vi "Timer Status.vi"(8 "error in":errorcluster, 9 "Position Correct?":bool, 10 "Step Status":string, 11 "Car Wash Steps":string[][](array[string])) -> (0 "error out":errorcluster, 2 "Timer Control":T1=enum."Start", 3 "Time Target":dbl, 5 "New Step Status":string)   [LabVIEW 2020]
uses:
  Timer Controls.ctl
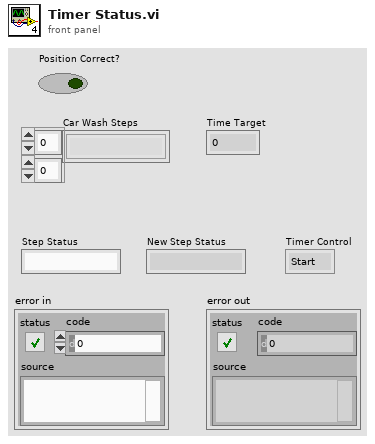
[diagram p1: front panel]
types:
  T1 = typedef "Timer Controls.ctl" = enum16{"Reset", "Start", "Stop"}
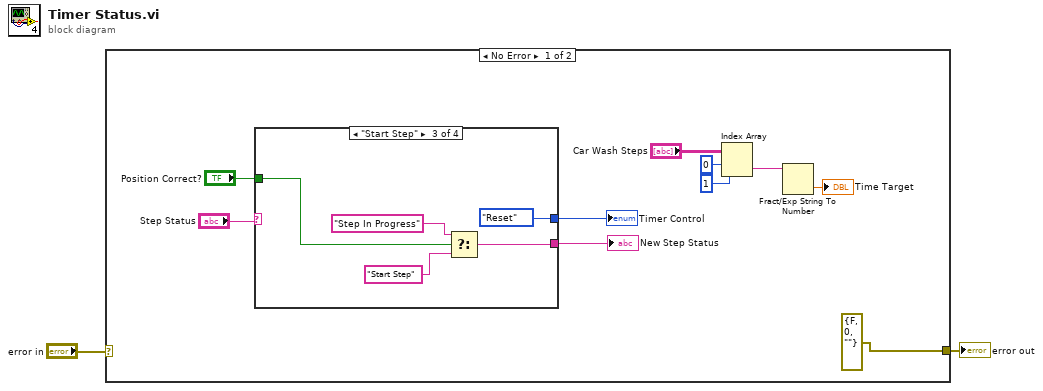
[diagram p0: block diagram]
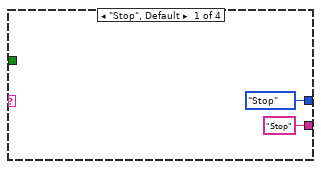
[diagram p2: hidden frame]
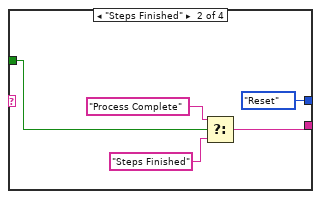
[diagram p3: hidden frame]
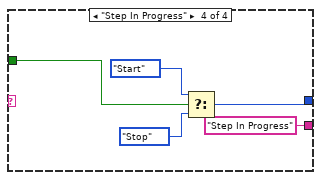
[diagram p4: hidden frame]
diagram:
  n1 = case shown="No Error" "error in" {
    selector: "error in" -> [_ w30]
    tunnel: [errorcluster {"status"=FALSE, "code"=0, "source"=""} ("error IO") w30] -> w1
    frame No Error {
      n2 = case shown="\"Start Step\"" "Step Status" {
        tunnel: [Timer_Controls."Stop" ("Timer Control") Timer_Controls."Reset" ("Timer Control") Timer_Controls."Reset" ("Timer Control") w26] -> w4
        tunnel: ["Stop" ("New Step Status") w17 w21 "Step In Progress" ("New Step Status")] -> w7
        tunnel: "Position Correct?" -> [_ w18 w23 w25]
        frame "Stop", Default {
        }
        frame "Steps Finished" {
          n3 = Select(t="Process Complete" ("New Step Status"), s=w18, f="Steps Finished" ("New Step Status")) -> (s? t:f=w17:string)
        }
        frame "Start Step" {
          n4 = Select(t="Step In Progress" ("New Step Status"), s=w23, f="Start Step" ("New Step Status")) -> (s? t:f=w21:string)
        }
        frame "Step In Progress" {
          n5 = Select(t=Timer_Controls."Start" ("Timer Control"), s=w25, f=Timer_Controls."Stop" ("Timer Control")) -> (s? t:f=w26:T1)
        }
      }
      "New Step Status" <- w7
      "Timer Control" <- w4
      n6 = Index Array(array="Car Wash Steps", index (row)=0, index (col)=1 ("disabled index (col)")) -> (element=w11:string)
      n7 = Fract/Exp String To Number(string=w11) -> (number=→"Time Target":dbl)  [unwired: 3 in, 1 out]
    }
    frame Error {
    }
  }
  "error out" <- w1
